vi "Enqueue Return Value.vi"(8 "error in (no error)":errorcluster, 10 "Indicator Values":cluster{"Name":string, "Variant Data":variant}[](array[cluster]), 11 "Mock In":refnum<class "Responsive Mock.lvclass">) -> (0 "error out":errorcluster, 3 "Mock Out":refnum<class "Responsive Mock.lvclass">)   [LabVIEW 2020, in "Responsive Mock.lvclass"]
uses:
  Responsive Mock.lvclass
  Responsive Mock.lvclass/Responsive Mock.ctl
  Core/VI Call/VI Call.lvclass
  Parametric VI Call/Parametric VI Call.lvclass
  C:/git/astemes-lmock/source/Core/VI Call/VI Call.lvclass
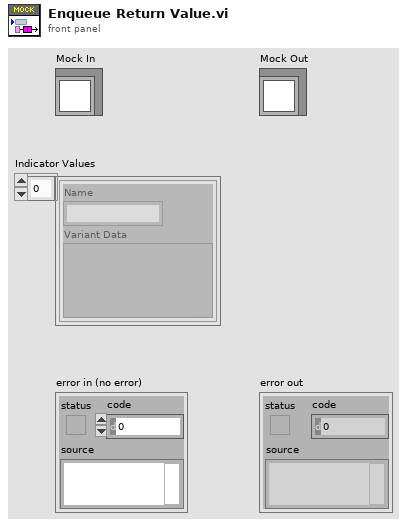
[diagram p1: front panel]
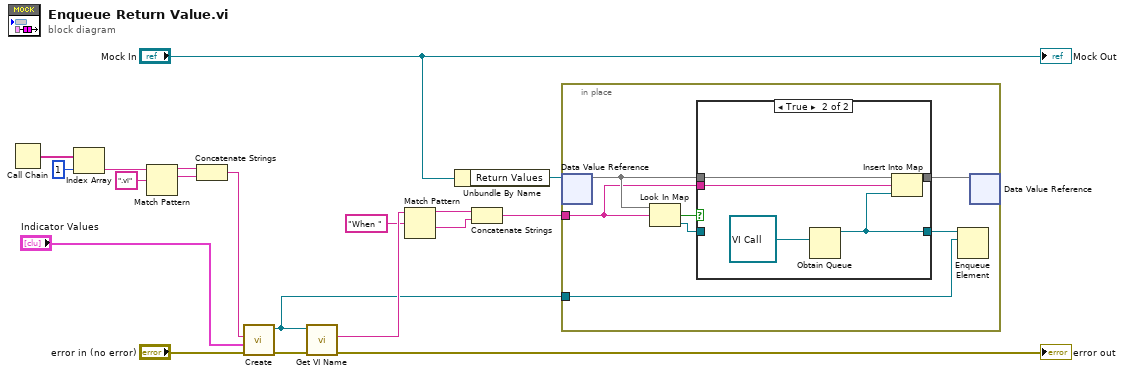
[diagram p0: block diagram]
diagram:
  n1 = Call Chain() -> (call chain=w8:string[])
  n2 = Index Array(array=w8, index=1) -> (element=w3:string)
  n3 = Match Pattern(string=w3, regular expression=".vi") -> (before substring=w5:string, match substring=w4:string)  [unwired: 1 in, 2 out]
  n4 = Concatenate Strings(w5, w4) -> (w1:string)
  n5 = call "Create.vi"("error in (no error)"="error in (no error)", "Control Values"="Indicator Values", "VI Name"=w1) -> ("error out"=w18:errorcluster, "Parametric VI Call Out"=w9:refnum<class "Parametric VI Call.lvclass">)  [unwired: 7 in]
  n6 = call-dynamic "Get VI Name.vi"("error in (no error)"=w18, "Parametric VI Call In"=w9) -> ("error out"=→"error out":errorcluster, "VI Name"=w16:string)  [unwired: 8 in]
  n7 = Match Pattern(string=w16, regular expression="When ") -> (before substring=w14:string, after substring=w13:string)  [unwired: 1 in, 2 out]
  n8 = Unbundle By Name("Mock In") -> ("Return Values"=w11:refnum<data-value>)
  n9 = Concatenate Strings(w14, w13) -> (w10:string)
  n10 = in-place {
    in-place-border: w10 -> [w23]
    in-place-border: w9 -> [w20]
    n11 = in-place-dvr #1(w11) -> (w25:map{string, refnum<queue>})  [unwired: 1 out]
    n12 = Look In Map(map=w25, key=w23) -> (key not found?=w26:bool, value=w24:refnum<queue>)  [unwired: 1 in]
    n13 = case shown="True" w26 {
      tunnel: w25 -> [w28 w32]
      tunnel: w24 -> [w27 _]
      tunnel: w23 -> [_ w31]
      tunnel: [w28 w30] -> w22
      tunnel: [w27 w29] -> w21
      frame False {
      }
      frame True {
        n14 = Obtain Queue(element data type=refnum<class "VI Call.lvclass"> refnum ("Call Out")) -> (queue out=w29:refnum<queue>)  [unwired: 4 in, 2 out]
        n15 = Insert Into Map(map in=w32, key=w31, value=w29) -> (map out=w30:map{string, refnum<queue>})  [unwired: 2 out]
      }
    }
    n16 = Enqueue Element(queue=w21, element=w20) -> ()  [unwired: 2 in, 3 out]
    n17 = in-place-dvr #1(w22) -> ()  [unwired: 2 out]
  }
  "Mock Out" <- "Mock In"
